vi "Export_fileName v10.6.0.vi"(0 "ITC503 Current Values":T2 {"ITC503 Gradient" format="%.2f"; "ITC503 Setpoint" min=-273.0 max=300000.0 step=0.0001 format="%.1f"; "ITC503 I" format="%_1f"; "ITC503 P" format="%_1f"; "ITC503 Temperature" min=0.0 max=1645.0 step=1e-05 format="%.2f"; "ITC503 Heater" min=0.0 max=100.0 step=0.01 scale=0.0..100.0}, 1 "iHR Current Values":T3={"iHR 550 Front Entrance"=0.0, "iHR550 Side Exit"=0.0, "iHR550 Wavelength"=897.9988, "iHR550 Exit Mirror"=2, "iHR550 Grating"="1", "Grating Index"=1} {"iHR550 Exit Mirror" items=["EntranceMirror", "ExitMirror", "Front", "Side"]}, 2 "Spectra Settings":T1={"Integration Time"=10.0, "Repetitions"=10, "Mapping Spectra"=TRUE} caption="Mapping Spectra Settings" {"Repetitions" min=1 max=100 step=1; "Integration Time" min=0.5 max=6000.0 step=1.0 format="%.1f"}, 3 "Drive Current Values":T4 {"Drive Z Position" min=-273.0 max=300000.0 step=0.0001 format="%.3f"; "Drive Y Position" min=-273.0 max=300000.0 step=0.0001 format="%.3f"; "Drive X Position" min=-273.0 max=300000.0 step=0.0001 format="%.3f"}) -> (5 "Filename":string)   [LabVIEW 2010]
uses:
  NPC3SG/TypeDefs/NPC3SG Current Values.ctl
  iHR550/TypeDefs/iHR Current Values.ctl
  ITC503/TypeDefs/ITC503 Current Values.ctl
  Mapping/TypeDefs/Mapping Spectra Params.ctl
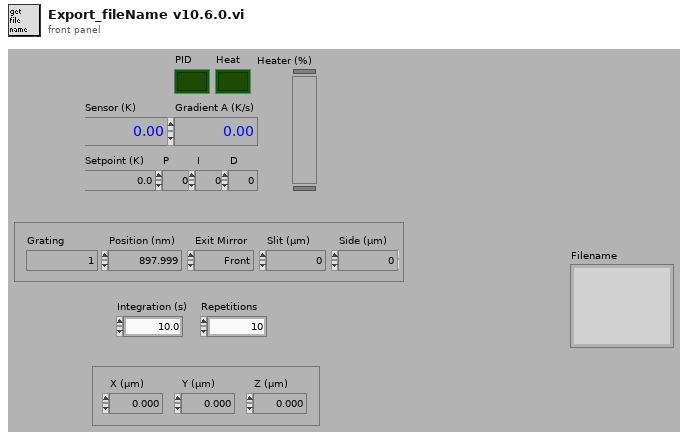
[diagram p1: front panel]
types:
  T1 = typedef "Mapping Spectra Params.ctl" = cluster{"Integration Time":dbl, "Repetitions":u16, "Mapping Spectra":bool}
  T2 = typedef "ITC503 Current Values.ctl" = cluster{"ITC503 Heater":dbl, "ITC503 Temperature":dbl, "ITC503 P":dbl, "ITC503 I":dbl, "ITC503 D":dbl, "ITC503 Setpoint":dbl, "ITC503 Gradient":dbl, "ITC503 Heater Auto":bool, "ITC503 PID Auto":bool}
  T3 = typedef "iHR Current Values.ctl" = cluster{"iHR 550 Front Entrance":dbl, "iHR550 Side Exit":dbl, "iHR550 Wavelength":dbl, "iHR550 Exit Mirror":i32, "iHR550 Grating":string, "Grating Index":i32}
  T4 = typedef "NPC3SG Current Values.ctl" = cluster{"Drive X Position":dbl, "Drive Y Position":dbl, "Drive Z Position":dbl}
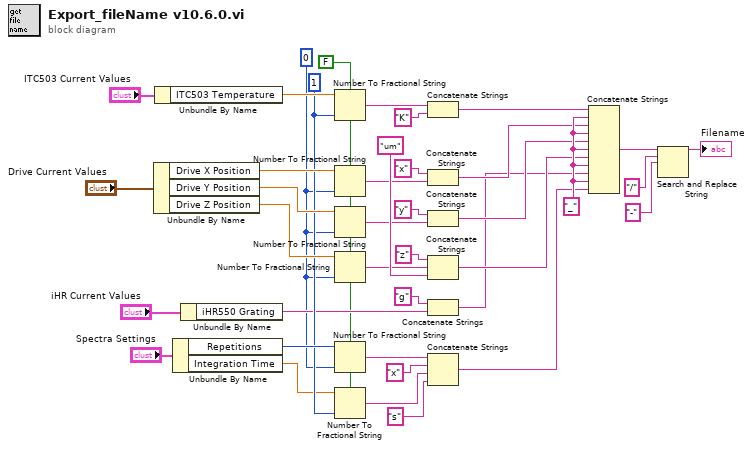
[diagram p0: block diagram]
diagram:
  w6 = i16 0 ("Genauigkeit (6)")
  w8 = "_" ("String")
  w7 = FALSE ("Systemdezimalzeichen verwenden (T)")
  w30 = i16 1 ("Genauigkeit (6)")
  n1 = Unbundle By Name("Drive Current Values") -> ("Drive X Position"=w33:dbl, "Drive Y Position"=w32:dbl, "Drive Z Position"=w31:dbl)
  n2 = Unbundle By Name("ITC503 Current Values") -> ("ITC503 Temperature"=w35:dbl)
  n3 = Unbundle By Name("Spectra Settings") -> ("Repetitions"=w34:u16, "Integration Time"=w23:dbl)
  n4 = Unbundle By Name("iHR Current Values") -> ("iHR550 Grating"=w14:string)
  n5 = Number To Fractional String(use system decimal point (T)=w7, number=w35, precision (6)=w30) -> (F-format string=w29:string)  [unwired: 1 in]
  n6 = Number To Fractional String(use system decimal point (T)=w7, number=w33, precision (6)=w6) -> (F-format string=w21:string)  [unwired: 1 in]
  n7 = Number To Fractional String(use system decimal point (T)=w7, number=w32, precision (6)=w6) -> (F-format string=w20:string)  [unwired: 1 in]
  n8 = Number To Fractional String(use system decimal point (T)=w7, number=w31, precision (6)=w6) -> (F-format string=w19:string)  [unwired: 1 in]
  n9 = Number To Fractional String(use system decimal point (T)=w7, number=w34, precision (6)=w6) -> (F-format string=w26:string)  [unwired: 1 in]
  n10 = Number To Fractional String(use system decimal point (T)=w7, number=w23, precision (6)=w30) -> (F-format string=w25:string)  [unwired: 1 in]
  n11 = Concatenate Strings(w29, "K" ("String")) -> (w13:string)
  n12 = Concatenate Strings("x" ("String"), w21) -> (w4:string)
  n13 = Concatenate Strings("y" ("String"), w20) -> (w3:string)
  n14 = Concatenate Strings("z" ("String"), w19, "um" ("String")) -> (w2:string)
  n15 = Concatenate Strings("g" ("String"), w14) -> (w1:string)
  n16 = Concatenate Strings(w26, "x" ("String"), w25, "s" ("String")) -> (w5:string)
  n17 = Concatenate Strings(w13, w8, w4, w8, w3, w8, w2, w8, w1, w8, w5) -> (w12:string)
  n18 = Search and Replace String(input string=w12, search string="/" ("Such-String"), replace string="-" ("replace string (\"\")")) -> (result string=→"Filename":string)  [unwired: 5 in, 3 out]
